vi "Update Engine.vi"(8 "error in (no error)":errorcluster, 10 "tdms file":refnum<k34>, 11 "Abstract Engine":refnum<class "Abstract Engine.lvclass">) -> (0 "error out":errorcluster, 3 "Abstract Engine out":refnum<class "Abstract Engine.lvclass">)   [LabVIEW 2025, in "Abstract Engine.lvlib" / "Abstract Engine.lvclass"]
uses:
  Abstract Engine.lvclass
  Abstract Instrument/Abstract Instrument.lvclass
  Abstract Engine.lvclass/Abstract Engine.ctl
  Read Engine Cluster.vi
  Users/Public/Documents/Sandia National Labs/TSS Plugin/CEF.lvlibp/Node/ReadChildren.vi
  Users/Public/Documents/Sandia National Labs/TSS Plugin/CEF.lvlibp/Node/CEF_Node.lvclass
  Users/Public/Documents/Sandia National Labs/TSS Plugin/CEF.lvlibp
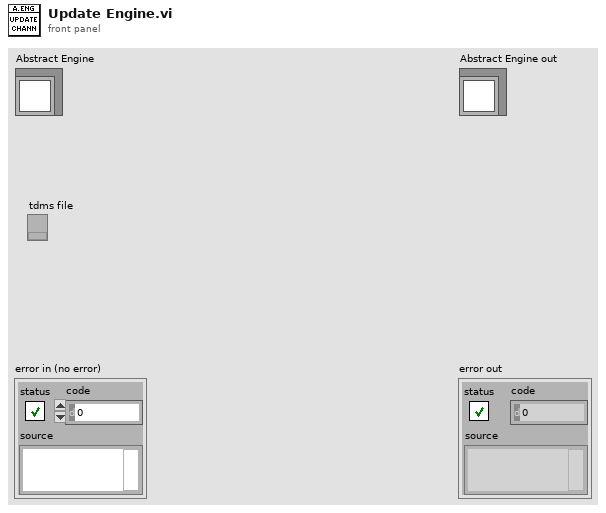
[diagram p1: front panel]
types:
  T1 = typedef "Abstract Engine.lvlib/Abstract Engine.lvclass/Engine Cluster.ctl" = cluster{"IP Address":string, "Type":string, "Initialized":bool, "InstrumentMap":map{string, cluster{"Initialized":bool, "Channels":T2[]}}}
  T2 = typedef "Abstract Engine.lvlib/Abstract Instrument.lvclass/Channel.ctl" = cluster{"Alias":string, "DataType":enum16{"Anaolg Input", "Waveform"}, "Unit":enum16{"---", "V", "A", "Ohm", "Hz", "uF", "degC", "deg"}, "Upper limit":dbl, "Lower limit":dbl, "Measurement":variant}
  T3 = map{string, cluster{"Initialized":bool, "Channels":T2[]}}
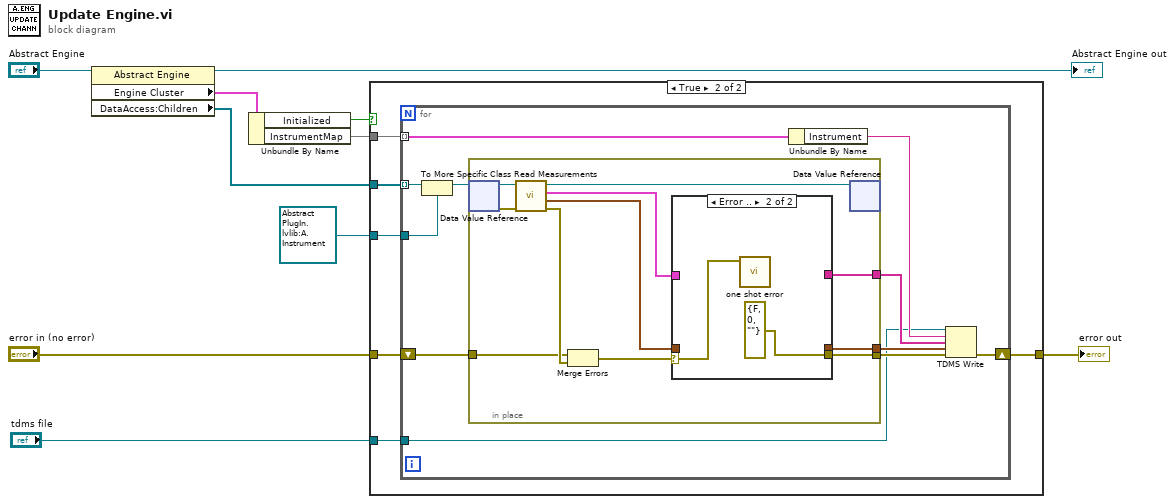
[diagram p0: block diagram]
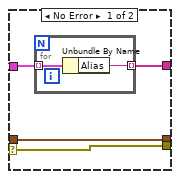
[diagram p3: hidden frame]
diagram:
  n1 = property class="Abstract Engine"(reference="Abstract Engine") -> (reference out=→"Abstract Engine out":refnum<class "Abstract Engine.lvclass">, "Engine Cluster"=w7:T1, "DataAccess:Children"=w9:refnum<data-value>[])  [unwired: 1 in, 1 out]
  n2 = Unbundle By Name(w7) -> ("Initialized"=w8:bool, "InstrumentMap"=w3:T3)
  n3 = case shown="True" w8 {
    tunnel: w9 -> [_ w17]
    tunnel: "error in (no error)" -> [w11 w16]
    tunnel: [w11 w15] -> w5
    tunnel: "tdms file" -> [_ w14]
    tunnel: w3 -> [_ w13]
    tunnel: refnum<data-value> refnum ("data value reference") -> [_ w12]
    frame False {
    }
    frame True {
      n4 = for {
        tunnel: w17 -> [w28] mode=indexing
        shift-right: [w24] -> w15
        shift-left: w16 -> [w26]
        tunnel: w14 -> [w18]
        tunnel: w13 -> [w22] mode=indexing
        tunnel: w12 -> [w19]
        n5 = To More Specific Class(target class=w19, reference=w28) -> (specific class reference=w27:refnum<data-value>)  [unwired: 1 in, 1 out]
        n6 = in-place {
          in-place-border: w26 -> [w35]
          in-place-border: [w29] -> w25
          in-place-border: [w33] -> w23
          in-place-border: [w30] -> w20
          n7 = in-place-dvr #1(w27) -> (w39:refnum<class "Abstract Instrument.lvclass">, w37:errorcluster)
          n8 = call-dynamic "Read Measurements.vi"("error in (no error)"=w37, "Abs Instrument in"=w39) -> ("error out"=w36:errorcluster, "Waveforms"=w31:waveform(dbl)[], "Measurements"=w34:T2[], "Abs Instrument out"=w38:refnum<class "Abstract Instrument.lvclass">)  [unwired: 6 in]
          n9 = Merge Errors(w35, w36) -> (w32:errorcluster)
          n10 = case shown="Error .." w32 {
            selector: w32 -> [w40 w47]
            tunnel: w34 -> [w43 _]
            tunnel: [w42 _] -> w33
            tunnel: w31 -> [w41 _]
            tunnel: [w41 _] -> w30
            tunnel: [w40 errorcluster {"status"=FALSE, "code"=0, "source"=""} ("error IO")] -> w29
            frame No Error {
              n11 = for {
                tunnel: w43 -> [w45] mode=indexing
                tunnel: [w44] -> w42 mode=indexing
                n12 = Unbundle By Name(w45) -> ("Alias"=w44:string)
              }
            }
            frame Error {
              n13 = call "one shot error.vi"("error in"=w47) -> ()  [unwired: 11 in]
            }
          }
          n14 = in-place-dvr #1(w38) -> ()  [unwired: 2 out]
        }
        n15 = Unbundle By Name(w22) -> ("Instrument"=w21:string)
        n16 = TDMS Write(0:w18, 5:w21, 7:w23, 9:w20, 11:w25) -> (15:w24:errorcluster)  [unwired: 1 in, 3 out]
      }
    }
  }
  "error out" <- w5
